vi "System Status.vi"(7 "Box ID":u8, 8 "error in (no error)":errorcluster, 11 "ENET in":refnum<class "ENET_BS120x.lvclass">) -> (0 "error out":errorcluster, 2 "Status":T1, 3 "ENET out":refnum<class "ENET_BS120x.lvclass">)   [LabVIEW 2021, in "BS120x Driver.lvlib" / "ENET_BS120x.lvclass"]
uses:
  ENET_BS120x.lvclass
  TypeDefs/System Status.ctl
  BS120x.lvclass
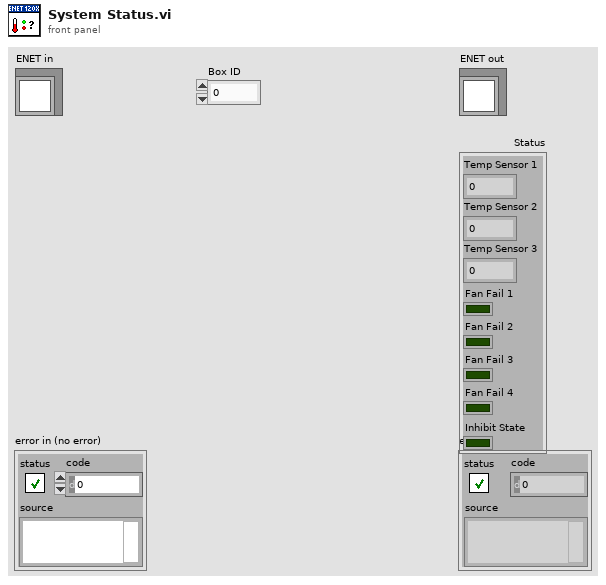
[diagram p1: front panel]
types:
  T1 = typedef "BS120x Driver.lvlib/BS120x.lvclass/System Status.ctl" = cluster{"Temp Sensor 1":dbl, "Temp Sensor 2":dbl, "Temp Sensor 3":dbl, "Fan Fail 1":bool, "Fan Fail 2":bool, "Fan Fail 3":bool, "Fan Fail 4":bool, "Inhibit State":bool}
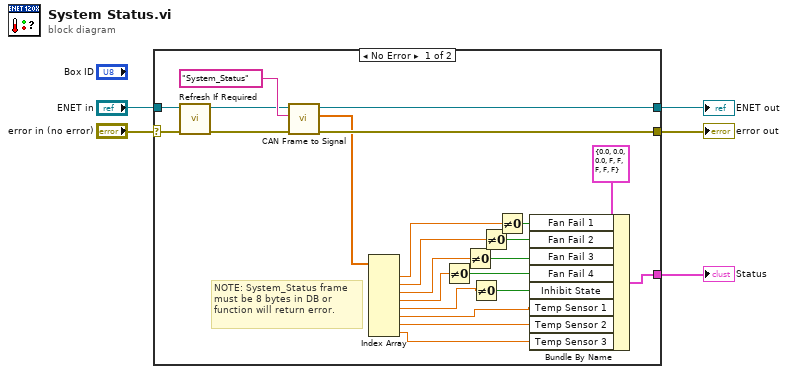
[diagram p0: block diagram]
diagram:
  n1 = case shown="No Error" "error in (no error)" {
    selector: "error in (no error)" -> [w14 w30]
    tunnel: [w28 w30] -> w5
    tunnel: [w16 w29] -> w4
    tunnel: [w15 _] -> w3
    tunnel: "ENET in" -> [w12 w29]
    frame No Error {
      # "NOTE: System_Status frame must be 8 bytes in DB or function will return error."
      n2 = call "Refresh If Required.vi"("error in (no error)"=w14, "Ethernet in"=w12) -> ("error out"=w13:errorcluster, "Ethernet out"=w11:refnum<class "ENET_BS120x.lvclass">)  [unwired: 8 in]
      n3 = call "CAN Frame to Signal.vi"("error in (no error)"=w13, "Frame"="System_Status" ("name"), "ENET in"=w11) -> ("error out"=w28:errorcluster, "signal data"=w17:dbl[], "ENET out"=w16:refnum<class "ENET_BS120x.lvclass">)  [unwired: 6 in]
      n4 = Index Array(array=w17) -> (element #1=w22:dbl, element #2=w23:dbl, element #3=w24:dbl, element #4=w25:dbl, element #5=w9:dbl, element #6=w8:dbl, element #7=w7:dbl, element #8=w6:dbl)  [unwired: 8 in]
      n5 = Not Equal To 0?(x=w25) -> (x != 0?=w20:bool)
      n6 = Not Equal To 0?(x=w24) -> (x != 0?=w21:bool)
      n7 = Not Equal To 0?(x=w9) -> (x != 0?=w10:bool)
      n8 = Not Equal To 0?(x=w23) -> (x != 0?=w19:bool)
      n9 = Not Equal To 0?(x=w22) -> (x != 0?=w18:bool)
      n10 = Bundle By Name(cluster=T1 {"Temp Sensor 1"=0.0, "Temp Sensor 2"=0.0, "Temp Sensor 3"=0.0, "Fan Fail 1"=FALSE, "Fan Fail 2"=FALSE, "Fan Fail 3"=FALSE, "Fan Fail 4"=FALSE, "Inhibit State"=FALSE} ("Status"), "Fan Fail 1"=w18, "Fan Fail 2"=w19, "Fan Fail 3"=w21, "Fan Fail 4"=w20, "Inhibit State"=w10, "Temp Sensor 1"=w8, "Temp Sensor 2"=w7, "Temp Sensor 3"=w6) -> (w15:T1)
    }
    frame Error {
    }
  }
  "error out" <- w5
  "ENET out" <- w4
  "Status" <- w3
